vi "Core Listen.vi"(8 "error in (no error)":errorcluster, 11 "CIFTemplateNode in":refnum<class "CIFCorePlugin.lvclass">) -> (0 "error out":errorcluster, 3 "CIFTemplateNode out":refnum<class "CIFCorePlugin.lvclass">)   [LabVIEW 2021, in "CIFCorePlugin.lvclass"]
uses:
  CIFCorePlugin.lvclass
  Typedef/Energized States.ctl
  CIFCorePlugin.lvclass/CIFCorePlugin.ctl
  CIFUtilities/CIFOutOfBand/CIFOutOfBand.lvclass/CIFOutOfBand.ctl
  CIFCoreOOB/OOB_Tx/Send/Update Status Command.vi
  CIFCoreOOB/OOB_Tx/Send/Update Override Command.vi
  CIFCoreOOB/OOB_Rx/Receive/Check for OOB Commands.vi
  CIFCoreOOB/OOB_Rx/Receive/Read FTE.vi
  Accessors/Timestamps/trash_Write FTE.vi
  SubVIs/Refresh Stats.vi
  CIFUtilities/CIFOutOfBand/Write OOB DVR.vi
  CIFUtilities/CIFOutOfBand/Utilities/Command to Bitwise Command.vi
  CIFUtilities/CIFOutOfBand/Accessors/Read Local OOB Data.vi
  CIFUtilities/CIFOutOfBand/Accessors/Write Local OOB Data.vi
  CIFUtilities/CIFOutOfBand/Read OOB DVR.vi
  CIFCoreOOB/OOB_Rx/Private/Command Settings.vi
  CIFCoreOOB/OOB_Rx/Private/Read Payload.vi
  CIFCoreOOB/OOB_Tx/CIFCoreOOB_Tx.lvclass
  D:/dev/CIF-LVCore/src/CIFUtilities/CIFOutOfBand/CIFOutOfBand.lvclass
  CIFCoreOOB/OOB_Rx/CIFCoreOOB_Rx.lvclass
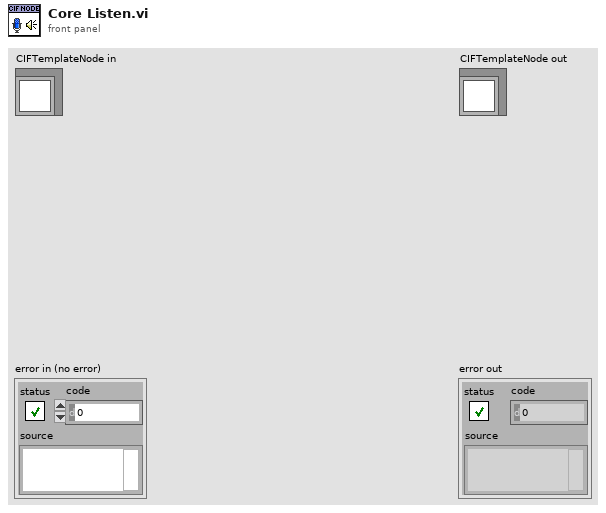
[diagram p1: front panel]
types:
  T1 = typedef "CIFCorePlugin.lvclass/Energized States.ctl" = enum16{"Listen", "Prepare", "Execute", "Housekeep", "Cleanup", "Destroy"}
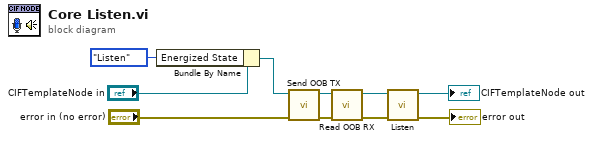
[diagram p0: block diagram]
diagram:
  n1 = Bundle By Name(cluster="CIFTemplateNode in", "Energized State"=Energized_States."Listen") -> (w1:refnum<class "CIFCorePlugin.lvclass">)
  n2 = call "Send OOB TX.vi"("error in (no error)"="error in (no error)", "CIFCorePlugin in"=w1) -> ("error out"=w5:errorcluster, "CIFCorePlugin out"=w6:refnum<class "CIFCorePlugin.lvclass">)  [unwired: 8 in]
  n3 = call "Read OOB RX.vi"("error in (no error)"=w5, "CIFCorePlugin in"=w6) -> ("error out"=w9:errorcluster, "CIFCorePlugin out"=w4:refnum<class "CIFCorePlugin.lvclass">)  [unwired: 8 in]
  n4 = call-dynamic "Listen.vi"("error in (no error)"=w9, "CIFTemplateNode in"=w4) -> ("error out"=→"error out":errorcluster, "CIFTemplateNode out"=→"CIFTemplateNode out":refnum<class "CIFCorePlugin.lvclass">)  [unwired: 8 in]
